vi "BuscarValores (SubVI).vi"(9 "=":string="1", 10 "Columna":string="POC", 11 "Tabla":string="Tabla1") -> (3 "String":string)   [LabVIEW 2012]
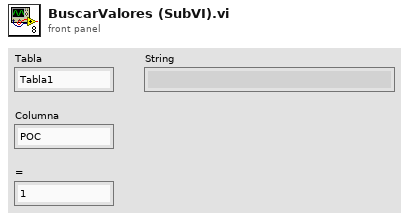
[diagram p1: front panel]
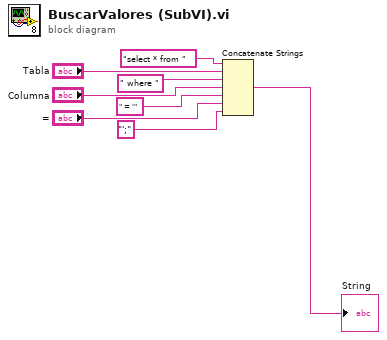
[diagram p0: block diagram]
diagram:
  n1 = Concatenate Strings("select * from " ("SQL query"), "Tabla", " where " ("string"), "Columna", " = '" ("Substring"), "=", "';") -> (→"String":string)
